vi "Log ERROR.vi"(7 "Logger Name":string, 8 "error in (no error)":errorcluster, 11 "Message":string) -> (0 "error out":errorcluster)   [LabVIEW 2020, in "Global_logger.lvlib"]
uses:
  Global_logger.lvlib
  Levels.ctl
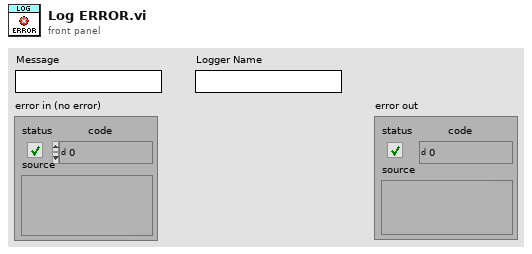
[diagram p1: front panel]
types:
  T1 = typedef "Global_logger.lvlib/Levels.ctl" = enum16{"ALL", "TRACE", "DEBUG", "INFO", "WARN", "ERROR", "FATAL", "OFF"}
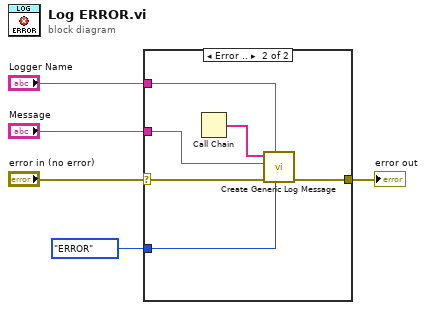
[diagram p0: block diagram]
diagram:
  n1 = case shown="Error .." "error in (no error)" {
    selector: "error in (no error)" -> [w6 w12]
    tunnel: [w6 w11] -> w4
    tunnel: "Message" -> [_ w10]
    tunnel: Levels."ERROR" ("Level") -> [_ w8]
    tunnel: "Logger Name" -> [_ w7]
    frame No Error {
    }
    frame Error {
      n2 = Call Chain() -> (call chain=w9:string[])
      n3 = call "Create Generic Log Message.vi"("Level"=w8, "Logger Name"=w7, "error in (no error)"=w12, "Message"=w10, "Call Chain"=w9) -> ("error out"=w11:errorcluster)  [unwired: 6 in]
    }
  }
  "error out" <- w4
